vi "Lab Panel V4.91.vi"() -> ()   [LabVIEW 2013] (continued)
                    n1115 = Unbundle(w2166) -> ("CYCLES"=w2157:dbl, "T-RISE mins"=w2163:dbl)  [unwired: 3 out]
                    n1116 = case shown="\"T-RISE TEST\"" w2164 {
                      tunnel: w2163 -> [_ _ w2173]
                      tunnel: [w2168 w2170 w2173] -> w2162
                      tunnel: w2157 -> [w2168 w2170 _]
                      tunnel: ["CHART PASS" "CYCLE PASS" "T-RISE PASS"] -> w2161
                      frame "CHART TEST", Default {
                      }
                      frame "CYCLE TEST" {
                      }
                      frame "T-RISE TEST" {
                      }
                    }
                    n1117 = Increment(x=w2157) -> (x+1=w2158:dbl)
                    n1118 = Greater Or Equal?(x=w2165, y=w2158) -> (x >= y?=w2167:bool)
                    n1119 = case shown="True" w2167 {
                      tunnel: w2162 -> [w2177 _]
                      tunnel: w2161 -> [w2176 _]
                      tunnel: w2160 -> [w2175 _]
                      tunnel: w2159 -> [w2174 _]
                      frame True {
                        n1120 = stacked-sequence {
                          tunnel: w2177 -> [w2181 _]
                          tunnel: w2176 -> [w2179 w2185]
                          tunnel: w2175 -> [_ w2188]
                          tunnel: w2174 -> [w2178 _]
                          frame #0 {
                            n1121 = Build Array(w2179) -> (w2182:string[])
                            n1122 = Build Array(w2181) -> (w2180:dbl[])
                            n1123 = TDMS Write(0:w2178, 5:"TEST PASS", 7:w2182, 9:w2180) -> (15:w2184:errorcluster)  [unwired: 2 in, 3 out]
                            n1124 = local write "data file error"(w2184) -> ()
                          }
                          frame #1 {
                            n1125 = Bundle(cluster=w2188, "STATUS"=w2185) -> (w2186:T4)  [unwired: 2 in]
                            n1126 = local write "RESULT LAB02-1"(TRUE) -> ()
                            n1127 = local write "DISP LAB02-1"(w2186) -> ()
                          }
                        }
                      }
                      frame False {
                      }
                    }
                  }
                }
              }
              frame #3 {
                # "LAB02-2"
                n1128 = Less?(x=w2189, y=2) -> (x < y?=w2192:bool)
                n1129 = local read "DISP LAB02-2"() -> (w2194:T4)
                n1130 = Unbundle(w2194) -> ("STATUS"=w2195:string)  [unwired: 2 out]
                n1131 = Equal?(x=w2195, y="RUN") -> (x = y?=w2191:bool)
                n1132 = And(x=w2191, y=w2192) -> (x .and. y?=w2190:bool)
                n1133 = case shown="True" w2190 {
                  tunnel: w2194 -> [_ w2200]
                  tunnel: w2189 -> [_ w2204]
                  frame False {
                  }
                  frame True {
                    n1134 = local read "SET LAB02-2"() -> (w2206:T5)
                    n1135 = local read "TDMS LAB02-2"() -> (w2199:refnum<k34>)
                    n1136 = Unbundle(w2200) -> ("CYCLE"=w2205:dbl)  [unwired: 2 out]
                    n1137 = Unbundle(w2206) -> ("CYCLES"=w2197:dbl, "T-RISE mins"=w2203:dbl)  [unwired: 3 out]
                    n1138 = case shown="\"T-RISE TEST\"" w2204 {
                      tunnel: w2203 -> [_ _ w2213]
                      tunnel: [w2208 w2210 w2213] -> w2202
                      tunnel: w2197 -> [w2208 w2210 _]
                      tunnel: ["CHART PASS" "CYCLE PASS" "T-RISE PASS"] -> w2201
                      frame "CHART TEST", Default {
                      }
                      frame "CYCLE TEST" {
                      }
                      frame "T-RISE TEST" {
                      }
                    }
                    n1139 = Increment(x=w2197) -> (x+1=w2198:dbl)
                    n1140 = Greater Or Equal?(x=w2205, y=w2198) -> (x >= y?=w2207:bool)
                    n1141 = case shown="True" w2207 {
                      tunnel: w2202 -> [w2217 _]
                      tunnel: w2201 -> [w2216 _]
                      tunnel: w2200 -> [w2215 _]
                      tunnel: w2199 -> [w2214 _]
                      frame True {
                        n1142 = stacked-sequence {
                          tunnel: w2217 -> [w2221 _]
                          tunnel: w2216 -> [w2219 w2225]
                          tunnel: w2215 -> [_ w2228]
                          tunnel: w2214 -> [w2218 _]
                          frame #0 {
                            n1143 = Build Array(w2219) -> (w2222:string[])
                            n1144 = Build Array(w2221) -> (w2220:dbl[])
                            n1145 = TDMS Write(0:w2218, 5:"TEST PASS", 7:w2222, 9:w2220) -> (15:w2224:errorcluster)  [unwired: 2 in, 3 out]
                            n1146 = local write "data file error"(w2224) -> ()
                          }
                          frame #1 {
                            n1147 = Bundle(cluster=w2228, "STATUS"=w2225) -> (w2226:T4)  [unwired: 2 in]
                            n1148 = local write "RESULT LAB02-2"(TRUE) -> ()
                            n1149 = local write "DISP LAB02-2"(w2226) -> ()
                          }
                        }
                      }
                      frame False {
                      }
                    }
                  }
                }
              }
              frame #4 {
                # "LAB03-1"
                n1150 = Less?(x=w2229, y=2) -> (x < y?=w2232:bool)
                n1151 = local read "DISP LAB03-1"() -> (w2234:T4)
                n1152 = Unbundle(w2234) -> ("STATUS"=w2235:string)  [unwired: 2 out]
                n1153 = Equal?(x=w2235, y="RUN") -> (x = y?=w2231:bool)
                n1154 = And(x=w2231, y=w2232) -> (x .and. y?=w2230:bool)
                n1155 = case shown="True" w2230 {
                  tunnel: w2234 -> [_ w2240]
                  tunnel: w2229 -> [_ w2244]
                  frame False {
                  }
                  frame True {
                    n1156 = local read "SET LAB03-1"() -> (w2246:T5)
                    n1157 = local read "TDMS LAB03-1"() -> (w2239:refnum<k34>)
                    n1158 = Unbundle(w2240) -> ("CYCLE"=w2245:dbl)  [unwired: 2 out]
                    n1159 = Unbundle(w2246) -> ("CYCLES"=w2237:dbl, "T-RISE mins"=w2243:dbl)  [unwired: 3 out]
                    n1160 = case shown="\"T-RISE TEST\"" w2244 {
                      tunnel: w2243 -> [_ _ w2253]
                      tunnel: [w2248 w2250 w2253] -> w2242
                      tunnel: w2237 -> [w2248 w2250 _]
                      tunnel: ["CHART PASS" "CYCLE PASS" "T-RISE PASS"] -> w2241
                      frame "CHART TEST", Default {
                      }
                      frame "CYCLE TEST" {
                      }
                      frame "T-RISE TEST" {
                      }
                    }
                    n1161 = Increment(x=w2237) -> (x+1=w2238:dbl)
                    n1162 = Greater Or Equal?(x=w2245, y=w2238) -> (x >= y?=w2247:bool)
                    n1163 = case shown="True" w2247 {
                      tunnel: w2242 -> [w2257 _]
                      tunnel: w2241 -> [w2256 _]
                      tunnel: w2240 -> [w2255 _]
                      tunnel: w2239 -> [w2254 _]
                      frame True {
                        n1164 = stacked-sequence {
                          tunnel: w2257 -> [w2261 _]
                          tunnel: w2256 -> [w2259 w2265]
                          tunnel: w2255 -> [_ w2268]
                          tunnel: w2254 -> [w2258 _]
                          frame #0 {
                            n1165 = Build Array(w2259) -> (w2262:string[])
                            n1166 = Build Array(w2261) -> (w2260:dbl[])
                            n1167 = TDMS Write(0:w2258, 5:"TEST PASS", 7:w2262, 9:w2260) -> (15:w2264:errorcluster)  [unwired: 2 in, 3 out]
                            n1168 = local write "data file error"(w2264) -> ()
                          }
                          frame #1 {
                            n1169 = Bundle(cluster=w2268, "STATUS"=w2265) -> (w2266:T4)  [unwired: 2 in]
                            n1170 = local write "RESULT LAB03-1"(TRUE) -> ()
                            n1171 = local write "DISP LAB03-1"(w2266) -> ()
                          }
                        }
                      }
                      frame False {
                      }
                    }
                  }
                }
              }
              frame #5 {
                # "LAB03-2"
                n1172 = Less?(x=w2269, y=2) -> (x < y?=w2272:bool)
                n1173 = local read "DISP LAB03-2"() -> (w2274:T4)
                n1174 = Unbundle(w2274) -> ("STATUS"=w2275:string)  [unwired: 2 out]
                n1175 = Equal?(x=w2275, y="RUN") -> (x = y?=w2271:bool)
                n1176 = And(x=w2271, y=w2272) -> (x .and. y?=w2270:bool)
                n1177 = case shown="True" w2270 {
                  tunnel: w2274 -> [_ w2280]
                  tunnel: w2269 -> [_ w2284]
                  frame False {
                  }
                  frame True {
                    n1178 = local read "SET LAB03-2"() -> (w2286:T5)
                    n1179 = local read "TDMS LAB03-2"() -> (w2279:refnum<k34>)
                    n1180 = Unbundle(w2280) -> ("CYCLE"=w2285:dbl)  [unwired: 2 out]
                    n1181 = Unbundle(w2286) -> ("CYCLES"=w2277:dbl, "T-RISE mins"=w2283:dbl)  [unwired: 3 out]
                    n1182 = case shown="\"T-RISE TEST\"" w2284 {
                      tunnel: w2283 -> [_ _ w2293]
                      tunnel: [w2288 w2290 w2293] -> w2282
                      tunnel: w2277 -> [w2288 w2290 _]
                      tunnel: ["CHART PASS" "CYCLE PASS" "T-RISE PASS"] -> w2281
                      frame "CHART TEST", Default {
                      }
                      frame "CYCLE TEST" {
                      }
                      frame "T-RISE TEST" {
                      }
                    }
                    n1183 = Increment(x=w2277) -> (x+1=w2278:dbl)
                    n1184 = Greater Or Equal?(x=w2285, y=w2278) -> (x >= y?=w2287:bool)
                    n1185 = case shown="True" w2287 {
                      tunnel: w2282 -> [w2297 _]
                      tunnel: w2281 -> [w2296 _]
                      tunnel: w2280 -> [w2295 _]
                      tunnel: w2279 -> [w2294 _]
                      frame True {
                        n1186 = stacked-sequence {
                          tunnel: w2297 -> [w2301 _]
                          tunnel: w2296 -> [w2299 w2305]
                          tunnel: w2295 -> [_ w2308]
                          tunnel: w2294 -> [w2298 _]
                          frame #0 {
                            n1187 = Build Array(w2299) -> (w2302:string[])
                            n1188 = Build Array(w2301) -> (w2300:dbl[])
                            n1189 = TDMS Write(0:w2298, 5:"TEST PASS", 7:w2302, 9:w2300) -> (15:w2304:errorcluster)  [unwired: 2 in, 3 out]
                            n1190 = local write "data file error"(w2304) -> ()
                          }
                          frame #1 {
                            n1191 = Bundle(cluster=w2308, "STATUS"=w2305) -> (w2306:T4)  [unwired: 2 in]
                            n1192 = local write "RESULT LAB03-2"(TRUE) -> ()
                            n1193 = local write "DISP LAB03-2"(w2306) -> ()
                          }
                        }
                      }
                      frame False {
                      }
                    }
                  }
                }
              }
              frame #6 {
                # "LAB04-1"
                n1194 = Less?(x=w2309, y=2) -> (x < y?=w2312:bool)
                n1195 = local read "DISP LAB04-1"() -> (w2314:T4)
                n1196 = Unbundle(w2314) -> ("STATUS"=w2315:string)  [unwired: 2 out]
                n1197 = Equal?(x=w2315, y="RUN") -> (x = y?=w2311:bool)
                n1198 = And(x=w2311, y=w2312) -> (x .and. y?=w2310:bool)
                n1199 = case shown="True" w2310 {
                  tunnel: w2314 -> [_ w2320]
                  tunnel: w2309 -> [_ w2324]
                  frame False {
                  }
                  frame True {
                    n1200 = local read "SET LAB04-1"() -> (w2326:T5)
                    n1201 = local read "TDMS LAB04-1"() -> (w2319:refnum<k34>)
                    n1202 = Unbundle(w2320) -> ("CYCLE"=w2325:dbl)  [unwired: 2 out]
                    n1203 = Unbundle(w2326) -> ("CYCLES"=w2317:dbl, "T-RISE mins"=w2323:dbl)  [unwired: 3 out]
                    n1204 = case shown="\"T-RISE TEST\"" w2324 {
                      tunnel: w2323 -> [_ _ w2333]
                      tunnel: [w2328 w2330 w2333] -> w2322
                      tunnel: w2317 -> [w2328 w2330 _]
                      tunnel: ["CHART PASS" "CYCLE PASS" "T-RISE PASS"] -> w2321
                      frame "CHART TEST", Default {
                      }
                      frame "CYCLE TEST" {
                      }
                      frame "T-RISE TEST" {
                      }
                    }
                    n1205 = Increment(x=w2317) -> (x+1=w2318:dbl)
                    n1206 = Greater Or Equal?(x=w2325, y=w2318) -> (x >= y?=w2327:bool)
                    n1207 = case shown="True" w2327 {
                      tunnel: w2322 -> [w2337 _]
                      tunnel: w2321 -> [w2336 _]
                      tunnel: w2320 -> [w2335 _]
                      tunnel: w2319 -> [w2334 _]
                      frame True {
                        n1208 = stacked-sequence {
                          tunnel: w2337 -> [w2341 _]
                          tunnel: w2336 -> [w2339 w2345]
                          tunnel: w2335 -> [_ w2348]
                          tunnel: w2334 -> [w2338 _]
                          frame #0 {
                            n1209 = Build Array(w2339) -> (w2342:string[])
                            n1210 = Build Array(w2341) -> (w2340:dbl[])
                            n1211 = TDMS Write(0:w2338, 5:"TEST PASS", 7:w2342, 9:w2340) -> (15:w2344:errorcluster)  [unwired: 2 in, 3 out]
                            n1212 = local write "data file error"(w2344) -> ()
                          }
                          frame #1 {
                            n1213 = Bundle(cluster=w2348, "STATUS"=w2345) -> (w2346:T4)  [unwired: 2 in]
                            n1214 = local write "RESULT LAB04-1"(TRUE) -> ()
                            n1215 = local write "DISP LAB04-1"(w2346) -> ()
                          }
                        }
                      }
                      frame False {
                      }
                    }
                  }
                }
              }
              frame #7 {
                # "LAB04-2"
                n1216 = Less?(x=w2349, y=2) -> (x < y?=w2352:bool)
                n1217 = local read "DISP LAB04-2"() -> (w2354:T4)
                n1218 = Unbundle(w2354) -> ("STATUS"=w2355:string)  [unwired: 2 out]
                n1219 = Equal?(x=w2355, y="RUN") -> (x = y?=w2351:bool)
                n1220 = And(x=w2351, y=w2352) -> (x .and. y?=w2350:bool)
                n1221 = case shown="True" w2350 {
                  tunnel: w2354 -> [_ w2360]
                  tunnel: w2349 -> [_ w2364]
                  frame False {
                  }
                  frame True {
                    n1222 = local read "SET LAB04-2"() -> (w2366:T5)
                    n1223 = local read "TDMS LAB04-2"() -> (w2359:refnum<k34>)
                    n1224 = Unbundle(w2360) -> ("CYCLE"=w2365:dbl)  [unwired: 2 out]
                    n1225 = Unbundle(w2366) -> ("CYCLES"=w2357:dbl, "T-RISE mins"=w2363:dbl)  [unwired: 3 out]
                    n1226 = case shown="\"T-RISE TEST\"" w2364 {
                      tunnel: w2363 -> [_ _ w2373]
                      tunnel: [w2368 w2370 w2373] -> w2362
                      tunnel: w2357 -> [w2368 w2370 _]
                      tunnel: ["CHART PASS" "CYCLE PASS" "T-RISE PASS"] -> w2361
                      frame "CHART TEST", Default {
                      }
                      frame "CYCLE TEST" {
                      }
                      frame "T-RISE TEST" {
                      }
                    }
                    n1227 = Increment(x=w2357) -> (x+1=w2358:dbl)
                    n1228 = Greater Or Equal?(x=w2365, y=w2358) -> (x >= y?=w2367:bool)
                    n1229 = case shown="True" w2367 {
                      tunnel: w2362 -> [w2377 _]
                      tunnel: w2361 -> [w2376 _]
                      tunnel: w2360 -> [w2375 _]
                      tunnel: w2359 -> [w2374 _]
                      frame True {
                        n1230 = stacked-sequence {
                          tunnel: w2377 -> [w2381 _]
                          tunnel: w2376 -> [w2379 w2385]
                          tunnel: w2375 -> [_ w2388]
                          tunnel: w2374 -> [w2378 _]
                          frame #0 {
                            n1231 = Build Array(w2379) -> (w2382:string[])
                            n1232 = Build Array(w2381) -> (w2380:dbl[])
                            n1233 = TDMS Write(0:w2378, 5:"TEST PASS", 7:w2382, 9:w2380) -> (15:w2384:errorcluster)  [unwired: 2 in, 3 out]
                            n1234 = local write "data file error"(w2384) -> ()
                          }
                          frame #1 {
                            n1235 = Bundle(cluster=w2388, "STATUS"=w2385) -> (w2386:T4)  [unwired: 2 in]
                            n1236 = local write "RESULT LAB04-2"(TRUE) -> ()
                            n1237 = local write "DISP LAB04-2"(w2386) -> ()
                          }
                        }
                      }
                      frame False {
                      }
                    }
                  }
                }
              }
              frame #8 {
                # "LAB05-1"
                n1238 = Less?(x=w2389, y=2) -> (x < y?=w2392:bool)
                n1239 = local read "DISP LAB05-1"() -> (w2394:T4)
                n1240 = Unbundle(w2394) -> ("STATUS"=w2395:string)  [unwired: 2 out]
                n1241 = Equal?(x=w2395, y="RUN") -> (x = y?=w2391:bool)
                n1242 = And(x=w2391, y=w2392) -> (x .and. y?=w2390:bool)
                n1243 = case shown="True" w2390 {
                  tunnel: w2394 -> [_ w2400]
                  tunnel: w2389 -> [_ w2404]
                  frame False {
                  }
                  frame True {
                    n1244 = local read "SET LAB05-1"() -> (w2406:T5)
                    n1245 = local read "TDMS LAB05-1"() -> (w2399:refnum<k34>)
                    n1246 = Unbundle(w2400) -> ("CYCLE"=w2405:dbl)  [unwired: 2 out]
                    n1247 = Unbundle(w2406) -> ("CYCLES"=w2397:dbl, "T-RISE mins"=w2403:dbl)  [unwired: 3 out]
                    n1248 = case shown="\"T-RISE TEST\"" w2404 {
                      tunnel: w2403 -> [_ _ w2413]
                      tunnel: [w2408 w2410 w2413] -> w2402
                      tunnel: w2397 -> [w2408 w2410 _]
                      tunnel: ["CHART PASS" "CYCLE PASS" "T-RISE PASS"] -> w2401
                      frame "CHART TEST", Default {
                      }
                      frame "CYCLE TEST" {
                      }
                      frame "T-RISE TEST" {
                      }
                    }
                    n1249 = Increment(x=w2397) -> (x+1=w2398:dbl)
                    n1250 = Greater Or Equal?(x=w2405, y=w2398) -> (x >= y?=w2407:bool)
                    n1251 = case shown="True" w2407 {
                      tunnel: w2402 -> [w2417 _]
                      tunnel: w2401 -> [w2416 _]
                      tunnel: w2400 -> [w2415 _]
                      tunnel: w2399 -> [w2414 _]
                      frame True {
                        n1252 = stacked-sequence {
                          tunnel: w2417 -> [w2421 _]
                          tunnel: w2416 -> [w2419 w2425]
                          tunnel: w2415 -> [_ w2428]
                          tunnel: w2414 -> [w2418 _]
                          frame #0 {
                            n1253 = Build Array(w2419) -> (w2422:string[])
                            n1254 = Build Array(w2421) -> (w2420:dbl[])
                            n1255 = TDMS Write(0:w2418, 5:"TEST PASS", 7:w2422, 9:w2420) -> (15:w2424:errorcluster)  [unwired: 2 in, 3 out]
                            n1256 = local write "data file error"(w2424) -> ()
                          }
                          frame #1 {
                            n1257 = Bundle(cluster=w2428, "STATUS"=w2425) -> (w2426:T4)  [unwired: 2 in]
                            n1258 = local write "RESULT LAB05-1"(TRUE) -> ()
                            n1259 = local write "DISP LAB05-1"(w2426) -> ()
                          }
                        }
                      }
                      frame False {
                      }
                    }
                  }
                }
              }
              frame #9 {
                # "LAB05-2"
                n1260 = Less?(x=w2429, y=2) -> (x < y?=w2432:bool)
                n1261 = local read "DISP LAB05-2"() -> (w2434:T4)
                n1262 = Unbundle(w2434) -> ("STATUS"=w2435:string)  [unwired: 2 out]
                n1263 = Equal?(x=w2435, y="RUN") -> (x = y?=w2431:bool)
                n1264 = And(x=w2431, y=w2432) -> (x .and. y?=w2430:bool)
                n1265 = case shown="True" w2430 {
                  tunnel: w2434 -> [_ w2440]
                  tunnel: w2429 -> [_ w2444]
                  frame False {
                  }
                  frame True {
                    n1266 = local read "SET LAB05-2"() -> (w2446:T5)
                    n1267 = local read "TDMS LAB05-2"() -> (w2439:refnum<k34>)
                    n1268 = Unbundle(w2440) -> ("CYCLE"=w2445:dbl)  [unwired: 2 out]
                    n1269 = Unbundle(w2446) -> ("CYCLES"=w2437:dbl, "T-RISE mins"=w2443:dbl)  [unwired: 3 out]
                    n1270 = case shown="\"T-RISE TEST\"" w2444 {
                      tunnel: w2443 -> [_ _ w2453]
                      tunnel: [w2448 w2450 w2453] -> w2442
                      tunnel: w2437 -> [w2448 w2450 _]
                      tunnel: ["CHART PASS" "CYCLE PASS" "T-RISE PASS"] -> w2441
                      frame "CHART TEST", Default {
                      }
                      frame "CYCLE TEST" {
                      }
                      frame "T-RISE TEST" {
                      }
                    }
                    n1271 = Increment(x=w2437) -> (x+1=w2438:dbl)
                    n1272 = Greater Or Equal?(x=w2445, y=w2438) -> (x >= y?=w2447:bool)
                    n1273 = case shown="True" w2447 {
                      tunnel: w2442 -> [w2457 _]
                      tunnel: w2441 -> [w2456 _]
                      tunnel: w2440 -> [w2455 _]
                      tunnel: w2439 -> [w2454 _]
                      frame True {
                        n1274 = stacked-sequence {
                          tunnel: w2457 -> [w2461 _]
                          tunnel: w2456 -> [w2459 w2465]
                          tunnel: w2455 -> [_ w2468]
                          tunnel: w2454 -> [w2458 _]
                          frame #0 {
                            n1275 = Build Array(w2459) -> (w2462:string[])
                            n1276 = Build Array(w2461) -> (w2460:dbl[])
                            n1277 = TDMS Write(0:w2458, 5:"TEST PASS", 7:w2462, 9:w2460) -> (15:w2464:errorcluster)  [unwired: 2 in, 3 out]
                            n1278 = local write "data file error"(w2464) -> ()
                          }
                          frame #1 {
                            n1279 = Bundle(cluster=w2468, "STATUS"=w2465) -> (w2466:T4)  [unwired: 2 in]
                            n1280 = local write "RESULT LAB05-2"(TRUE) -> ()
                            n1281 = local write "DISP LAB05-2"(w2466) -> ()
                          }
                        }
                      }
                      frame False {
                      }
                    }
                  }
                }
              }
            }
          }
          frame #5 {
            # "check if test cycles reached for temperature rise test"
            n1282 = stacked-sequence {
              tunnel: w2498 -> [_ _ _ _ _ _ _ _ _ _]
              tunnel: w2497 -> [_ _ _ _ _ _ _ _ _ _]
              tunnel: w2496 -> [_ _ _ _ _ _ _ _ _ _]
              tunnel: w2495 -> [_ _ _ _ _ _ _ _ _ _]
              tunnel: w2494 -> [_ _ _ _ _ _ _ _ _ _]
              tunnel: w2493 -> [_ _ _ _ _ _ _ _ _ _]
              tunnel: w2492 -> [_ _ _ _ _ _ _ _ _ _]
              tunnel: w2491 -> [_ _ _ _ _ _ _ _ _ _]
              tunnel: w2490 -> [_ _ _ _ _ _ _ _ _ _]
              tunnel: w2489 -> [_ _ _ _ _ _ _ _ _ _]
              tunnel: w2488 -> [w2504 _ _ _ _ _ _ _ _ _]
              tunnel: w2478 -> [w2499 _ _ _ _ _ _ _ _ _]
              tunnel: w2487 -> [_ w2530 _ _ _ _ _ _ _ _]
              tunnel: w2486 -> [_ _ w2560 _ _ _ _ _ _ _]
              tunnel: w2485 -> [_ _ _ w2590 _ _ _ _ _ _]
              tunnel: w2484 -> [_ _ _ _ w2620 _ _ _ _ _]
              tunnel: w2483 -> [_ _ _ _ _ w2650 _ _ _ _]
              tunnel: w2482 -> [_ _ _ _ _ _ w2680 _ _ _]
              tunnel: w2481 -> [_ _ _ _ _ _ _ w2710 _ _]
              tunnel: w2480 -> [_ _ _ _ _ _ _ _ w2740 _]
              tunnel: w2479 -> [_ _ _ _ _ _ _ _ _ w2770]
              tunnel: w2477 -> [_ w2529 _ _ _ _ _ _ _ _]
              tunnel: w2476 -> [_ _ w2559 _ _ _ _ _ _ _]
              tunnel: w2475 -> [_ _ _ w2589 _ _ _ _ _ _]
              tunnel: w2474 -> [_ _ _ _ w2619 _ _ _ _ _]
              tunnel: w2473 -> [_ _ _ _ _ w2649 _ _ _ _]
              tunnel: w2472 -> [_ _ _ _ _ _ w2679 _ _ _]
              tunnel: w2471 -> [_ _ _ _ _ _ _ w2709 _ _]
              tunnel: w2470 -> [_ _ _ _ _ _ _ _ w2739 _]
              tunnel: w2469 -> [_ _ _ _ _ _ _ _ _ w2769]
              frame #0 {
                # "LAB01-1"
                n1283 = Equal?(x=w2504, y=2) -> (x = y?=w2502:bool)
                n1284 = local read "DISP LAB01-1"() -> (w2505:T4)
                n1285 = Unbundle(w2505) -> ("STATUS"=w2506:string)  [unwired: 2 out]
                n1286 = Equal?(x=w2506, y="RUN") -> (x = y?=w2501:bool)
                n1287 = And(x=w2501, y=w2502) -> (x .and. y?=w2500:bool)
                n1288 = case shown="True" w2500 {
                  tunnel: w2505 -> [_ w2509]
                  tunnel: w2499 -> [_ w2512]
                  frame False {
                  }
                  frame True {
                    n1289 = local read "SET LAB01-1"() -> (w2511:T5)
                    n1290 = local read "TDMS LAB01-1"() -> (w2508:refnum<k34>)
                    n1291 = Unbundle(w2509) -> ("CYCLE"=w2513:dbl)  [unwired: 2 out]
                    n1292 = Unbundle(w2511) -> ("T-RISE mins"=w2510:dbl)  [unwired: 4 out]
                    n1293 = Greater Or Equal?(x=w2513, y=w2512) -> (x >= y?=w2514:bool)
                    n1294 = case shown="True" w2514 {
                      tunnel: w2510 -> [w2517 _]
                      tunnel: w2509 -> [w2516 _]
                      tunnel: w2508 -> [w2515 _]
                      frame True {
                        n1295 = stacked-sequence {
                          tunnel: w2517 -> [w2520 _]
                          tunnel: w2516 -> [_ w2525]
                          tunnel: w2515 -> [w2518 _]
                          frame #0 {
                            n1296 = Build Array("T-RISE") -> (w2522:string[])
                            n1297 = Build Array(w2520) -> (w2521:dbl[])
                            n1298 = TDMS Write(0:w2518, 5:"TEST PASS", 7:w2522, 9:w2521) -> (15:w2524:errorcluster)  [unwired: 2 in, 3 out]
                            n1299 = local write "data file error"(w2524) -> ()
                          }
                          frame #1 {
                            n1300 = Bundle(cluster=w2525, "STATUS"="T-RISE PASS") -> (w2527:T4)  [unwired: 2 in]
                            n1301 = local write "RESULT LAB01-1"(TRUE) -> ()
                            n1302 = local write "DISP LAB01-1"(w2527) -> ()
                          }
                        }
                      }
                      frame False {
                      }
                    }
                  }
                }
              }
              frame #1 {
                # "LAB01-2"
                n1303 = Equal?(x=w2530, y=2) -> (x = y?=w2533:bool)
                n1304 = local read "DISP LAB01-2"() -> (w2535:T4)
                n1305 = Unbundle(w2535) -> ("STATUS"=w2536:string)  [unwired: 2 out]
                n1306 = Equal?(x=w2536, y="RUN") -> (x = y?=w2532:bool)
                n1307 = And(x=w2532, y=w2533) -> (x .and. y?=w2531:bool)
                n1308 = case shown="True" w2531 {
                  tunnel: w2535 -> [_ w2539]
                  tunnel: w2529 -> [_ w2542]
                  frame False {
                  }
                  frame True {
                    n1309 = local read "SET LAB01-2"() -> (w2541:T5)
                    n1310 = local read "TDMS LAB01-2"() -> (w2538:refnum<k34>)
                    n1311 = Unbundle(w2539) -> ("CYCLE"=w2543:dbl)  [unwired: 2 out]
                    n1312 = Unbundle(w2541) -> ("T-RISE mins"=w2540:dbl)  [unwired: 4 out]
                    n1313 = Greater Or Equal?(x=w2543, y=w2542) -> (x >= y?=w2544:bool)
                    n1314 = case shown="True" w2544 {
                      tunnel: w2540 -> [w2547 _]
                      tunnel: w2539 -> [w2546 _]
                      tunnel: w2538 -> [w2545 _]
                      frame True {
                        n1315 = stacked-sequence {
                          tunnel: w2547 -> [w2550 _]
                          tunnel: w2546 -> [_ w2555]
                          tunnel: w2545 -> [w2548 _]
                          frame #0 {
                            n1316 = Build Array("T-RISE") -> (w2552:string[])
                            n1317 = Build Array(w2550) -> (w2551:dbl[])
                            n1318 = TDMS Write(0:w2548, 5:"TEST PASS", 7:w2552, 9:w2551) -> (15:w2554:errorcluster)  [unwired: 2 in, 3 out]
                            n1319 = local write "data file error"(w2554) -> ()
                          }
                          frame #1 {
                            n1320 = Bundle(cluster=w2555, "STATUS"="T-RISE PASS") -> (w2557:T4)  [unwired: 2 in]
                            n1321 = local write "RESULT LAB01-2"(TRUE) -> ()
                            n1322 = local write "DISP LAB01-2"(w2557) -> ()
                          }
                        }
                      }
                      frame False {
                      }
                    }
                  }
                }
              }
              frame #2 {
                # "LAB02-1"
                n1323 = Equal?(x=w2560, y=2) -> (x = y?=w2563:bool)
                n1324 = local read "DISP LAB02-1"() -> (w2565:T4)
                n1325 = Unbundle(w2565) -> ("STATUS"=w2566:string)  [unwired: 2 out]
                n1326 = Equal?(x=w2566, y="RUN") -> (x = y?=w2562:bool)
                n1327 = And(x=w2562, y=w2563) -> (x .and. y?=w2561:bool)
                n1328 = case shown="True" w2561 {
                  tunnel: w2565 -> [_ w2569]
                  tunnel: w2559 -> [_ w2572]
                  frame False {
                  }
                  frame True {
                    n1329 = local read "SET LAB02-1"() -> (w2571:T5)
                    n1330 = local read "TDMS LAB02-1"() -> (w2568:refnum<k34>)
                    n1331 = Unbundle(w2569) -> ("CYCLE"=w2573:dbl)  [unwired: 2 out]
                    n1332 = Unbundle(w2571) -> ("T-RISE mins"=w2570:dbl)  [unwired: 4 out]
                    n1333 = Greater Or Equal?(x=w2573, y=w2572) -> (x >= y?=w2574:bool)
                    n1334 = case shown="True" w2574 {
                      tunnel: w2570 -> [w2577 _]
                      tunnel: w2569 -> [w2576 _]
                      tunnel: w2568 -> [w2575 _]
                      frame True {
                        n1335 = stacked-sequence {
                          tunnel: w2577 -> [w2580 _]
                          tunnel: w2576 -> [_ w2585]
                          tunnel: w2575 -> [w2578 _]
                          frame #0 {
                            n1336 = Build Array("T-RISE") -> (w2582:string[])
                            n1337 = Build Array(w2580) -> (w2581:dbl[])
                            n1338 = TDMS Write(0:w2578, 5:"TEST PASS", 7:w2582, 9:w2581) -> (15:w2584:errorcluster)  [unwired: 2 in, 3 out]
                            n1339 = local write "data file error"(w2584) -> ()
                          }
                          frame #1 {
                            n1340 = Bundle(cluster=w2585, "STATUS"="T-RISE PASS") -> (w2587:T4)  [unwired: 2 in]
                            n1341 = local write "RESULT LAB02-1"(TRUE) -> ()
                            n1342 = local write "DISP LAB02-1"(w2587) -> ()
                          }
                        }
                      }
                      frame False {
                      }
                    }
                  }
                }
              }
              frame #3 {
                # "LAB02-2"
                n1343 = Equal?(x=w2590, y=2) -> (x = y?=w2593:bool)
                n1344 = local read "DISP LAB02-2"() -> (w2595:T4)
                n1345 = Unbundle(w2595) -> ("STATUS"=w2596:string)  [unwired: 2 out]
                n1346 = Equal?(x=w2596, y="RUN") -> (x = y?=w2592:bool)
                n1347 = And(x=w2592, y=w2593) -> (x .and. y?=w2591:bool)
                n1348 = case shown="True" w2591 {
                  tunnel: w2595 -> [_ w2599]
                  tunnel: w2589 -> [_ w2602]
                  frame False {
                  }
                  frame True {
                    n1349 = local read "SET LAB02-2"() -> (w2601:T5)
                    n1350 = local read "TDMS LAB02-2"() -> (w2598:refnum<k34>)
                    n1351 = Unbundle(w2599) -> ("CYCLE"=w2603:dbl)  [unwired: 2 out]
                    n1352 = Unbundle(w2601) -> ("T-RISE mins"=w2600:dbl)  [unwired: 4 out]
                    n1353 = Greater Or Equal?(x=w2603, y=w2602) -> (x >= y?=w2604:bool)
                    n1354 = case shown="True" w2604 {
                      tunnel: w2600 -> [w2607 _]
                      tunnel: w2599 -> [w2606 _]
                      tunnel: w2598 -> [w2605 _]
                      frame True {
                        n1355 = stacked-sequence {
                          tunnel: w2607 -> [w2610 _]
                          tunnel: w2606 -> [_ w2615]
                          tunnel: w2605 -> [w2608 _]
                          frame #0 {
                            n1356 = Build Array("T-RISE") -> (w2612:string[])
                            n1357 = Build Array(w2610) -> (w2611:dbl[])
                            n1358 = TDMS Write(0:w2608, 5:"TEST PASS", 7:w2612, 9:w2611) -> (15:w2614:errorcluster)  [unwired: 2 in, 3 out]
                            n1359 = local write "data file error"(w2614) -> ()
                          }
                          frame #1 {
                            n1360 = Bundle(cluster=w2615, "STATUS"="T-RISE PASS") -> (w2617:T4)  [unwired: 2 in]
                            n1361 = local write "RESULT LAB02-2"(TRUE) -> ()
                            n1362 = local write "DISP LAB02-2"(w2617) -> ()
                          }
                        }
                      }
                      frame False {
                      }
                    }
                  }
                }
              }
              frame #4 {
                # "LAB03-1"
                n1363 = Equal?(x=w2620, y=2) -> (x = y?=w2623:bool)
                n1364 = local read "DISP LAB03-1"() -> (w2625:T4)
                n1365 = Unbundle(w2625) -> ("STATUS"=w2626:string)  [unwired: 2 out]
                n1366 = Equal?(x=w2626, y="RUN") -> (x = y?=w2622:bool)
                n1367 = And(x=w2622, y=w2623) -> (x .and. y?=w2621:bool)
                n1368 = case shown="True" w2621 {
                  tunnel: w2625 -> [_ w2629]
                  tunnel: w2619 -> [_ w2632]
                  frame False {
                  }
                  frame True {
                    n1369 = local read "SET LAB03-1"() -> (w2631:T5)
                    n1370 = local read "TDMS LAB03-1"() -> (w2628:refnum<k34>)
                    n1371 = Unbundle(w2629) -> ("CYCLE"=w2633:dbl)  [unwired: 2 out]
                    n1372 = Unbundle(w2631) -> ("T-RISE mins"=w2630:dbl)  [unwired: 4 out]
                    n1373 = Greater Or Equal?(x=w2633, y=w2632) -> (x >= y?=w2634:bool)
                    n1374 = case shown="True" w2634 {
                      tunnel: w2630 -> [w2637 _]
                      tunnel: w2629 -> [w2636 _]
                      tunnel: w2628 -> [w2635 _]
                      frame True {
                        n1375 = stacked-sequence {
                          tunnel: w2637 -> [w2640 _]
                          tunnel: w2636 -> [_ w2645]
                          tunnel: w2635 -> [w2638 _]
                          frame #0 {
                            n1376 = Build Array("T-RISE") -> (w2642:string[])
                            n1377 = Build Array(w2640) -> (w2641:dbl[])
                            n1378 = TDMS Write(0:w2638, 5:"TEST PASS", 7:w2642, 9:w2641) -> (15:w2644:errorcluster)  [unwired: 2 in, 3 out]
                            n1379 = local write "data file error"(w2644) -> ()
                          }
                          frame #1 {
                            n1380 = Bundle(cluster=w2645, "STATUS"="T-RISE PASS") -> (w2647:T4)  [unwired: 2 in]
                            n1381 = local write "RESULT LAB03-1"(TRUE) -> ()
                            n1382 = local write "DISP LAB03-1"(w2647) -> ()
                          }
                        }
                      }
                      frame False {
                      }
                    }
                  }
                }
              }
              frame #5 {
                # "LAB03-2"
                n1383 = Equal?(x=w2650, y=2) -> (x = y?=w2653:bool)
                n1384 = local read "DISP LAB03-2"() -> (w2655:T4)
                n1385 = Unbundle(w2655) -> ("STATUS"=w2656:string)  [unwired: 2 out]
                n1386 = Equal?(x=w2656, y="RUN") -> (x = y?=w2652:bool)
                n1387 = And(x=w2652, y=w2653) -> (x .and. y?=w2651:bool)
                n1388 = case shown="True" w2651 {
                  tunnel: w2655 -> [_ w2659]
                  tunnel: w2649 -> [_ w2662]
                  frame False {
                  }
                  frame True {
                    n1389 = local read "SET LAB03-2"() -> (w2661:T5)
                    n1390 = local read "TDMS LAB03-2"() -> (w2658:refnum<k34>)
                    n1391 = Unbundle(w2659) -> ("CYCLE"=w2663:dbl)  [unwired: 2 out]
                    n1392 = Unbundle(w2661) -> ("T-RISE mins"=w2660:dbl)  [unwired: 4 out]
                    n1393 = Greater Or Equal?(x=w2663, y=w2662) -> (x >= y?=w2664:bool)
                    n1394 = case shown="True" w2664 {
                      tunnel: w2660 -> [w2667 _]
                      tunnel: w2659 -> [w2666 _]
                      tunnel: w2658 -> [w2665 _]
                      frame True {
                        n1395 = stacked-sequence {
                          tunnel: w2667 -> [w2670 _]
                          tunnel: w2666 -> [_ w2675]
                          tunnel: w2665 -> [w2668 _]
                          frame #0 {
                            n1396 = Build Array("T-RISE") -> (w2672:string[])
                            n1397 = Build Array(w2670) -> (w2671:dbl[])
                            n1398 = TDMS Write(0:w2668, 5:"TEST PASS", 7:w2672, 9:w2671) -> (15:w2674:errorcluster)  [unwired: 2 in, 3 out]
                            n1399 = local write "data file error"(w2674) -> ()
                          }
                          frame #1 {
                            n1400 = Bundle(cluster=w2675, "STATUS"="T-RISE PASS") -> (w2677:T4)  [unwired: 2 in]
                            n1401 = local write "RESULT LAB03-2"(TRUE) -> ()
                            n1402 = local write "DISP LAB03-2"(w2677) -> ()
                          }
                        }
                      }
                      frame False {
                      }
                    }
                  }
                }
              }
              frame #6 {
                # "LAB04-1"
                n1403 = Equal?(x=w2680, y=2) -> (x = y?=w2683:bool)
                n1404 = local read "DISP LAB04-1"() -> (w2685:T4)
                n1405 = Unbundle(w2685) -> ("STATUS"=w2686:string)  [unwired: 2 out]
                n1406 = Equal?(x=w2686, y="RUN") -> (x = y?=w2682:bool)
                n1407 = And(x=w2682, y=w2683) -> (x .and. y?=w2681:bool)
                n1408 = case shown="True" w2681 {
                  tunnel: w2685 -> [_ w2689]
                  tunnel: w2679 -> [_ w2692]
                  frame False {
                  }
                  frame True {
                    n1409 = local read "SET LAB04-1"() -> (w2691:T5)
                    n1410 = local read "TDMS LAB04-1"() -> (w2688:refnum<k34>)
                    n1411 = Unbundle(w2689) -> ("CYCLE"=w2693:dbl)  [unwired: 2 out]
                    n1412 = Unbundle(w2691) -> ("T-RISE mins"=w2690:dbl)  [unwired: 4 out]
                    n1413 = Greater Or Equal?(x=w2693, y=w2692) -> (x >= y?=w2694:bool)
                    n1414 = case shown="True" w2694 {
                      tunnel: w2690 -> [w2697 _]
                      tunnel: w2689 -> [w2696 _]
                      tunnel: w2688 -> [w2695 _]
                      frame True {
                        n1415 = stacked-sequence {
                          tunnel: w2697 -> [w2700 _]
                          tunnel: w2696 -> [_ w2705]
                          tunnel: w2695 -> [w2698 _]
                          frame #0 {
                            n1416 = Build Array("T-RISE") -> (w2702:string[])
                            n1417 = Build Array(w2700) -> (w2701:dbl[])
                            n1418 = TDMS Write(0:w2698, 5:"TEST PASS", 7:w2702, 9:w2701) -> (15:w2704:errorcluster)  [unwired: 2 in, 3 out]
                            n1419 = local write "data file error"(w2704) -> ()
                          }
                          frame #1 {
                            n1420 = Bundle(cluster=w2705, "STATUS"="T-RISE PASS") -> (w2707:T4)  [unwired: 2 in]
                            n1421 = local write "RESULT LAB04-1"(TRUE) -> ()
                            n1422 = local write "DISP LAB04-1"(w2707) -> ()
                          }
                        }
                      }
                      frame False {
                      }
                    }
                  }
                }
              }
              frame #7 {
                # "LAB04-2"
                n1423 = Equal?(x=w2710, y=2) -> (x = y?=w2713:bool)
                n1424 = local read "DISP LAB04-2"() -> (w2715:T4)
                n1425 = Unbundle(w2715) -> ("STATUS"=w2716:string)  [unwired: 2 out]
                n1426 = Equal?(x=w2716, y="RUN") -> (x = y?=w2712:bool)
                n1427 = And(x=w2712, y=w2713) -> (x .and. y?=w2711:bool)
                n1428 = case shown="True" w2711 {
                  tunnel: w2715 -> [_ w2719]
                  tunnel: w2709 -> [_ w2722]
                  frame False {
                  }
                  frame True {
                    n1429 = local read "SET LAB04-2"() -> (w2721:T5)
                    n1430 = local read "TDMS LAB04-2"() -> (w2718:refnum<k34>)
                    n1431 = Unbundle(w2719) -> ("CYCLE"=w2723:dbl)  [unwired: 2 out]
                    n1432 = Unbundle(w2721) -> ("T-RISE mins"=w2720:dbl)  [unwired: 4 out]
                    n1433 = Greater Or Equal?(x=w2723, y=w2722) -> (x >= y?=w2724:bool)
                    n1434 = case shown="True" w2724 {
                      tunnel: w2720 -> [w2727 _]
                      tunnel: w2719 -> [w2726 _]
                      tunnel: w2718 -> [w2725 _]
                      frame True {
                        n1435 = stacked-sequence {
                          tunnel: w2727 -> [w2730 _]
                          tunnel: w2726 -> [_ w2735]
                          tunnel: w2725 -> [w2728 _]
                          frame #0 {
                            n1436 = Build Array("T-RISE") -> (w2732:string[])
                            n1437 = Build Array(w2730) -> (w2731:dbl[])
                            n1438 = TDMS Write(0:w2728, 5:"TEST PASS", 7:w2732, 9:w2731) -> (15:w2734:errorcluster)  [unwired: 2 in, 3 out]
                            n1439 = local write "data file error"(w2734) -> ()
                          }
                          frame #1 {
                            n1440 = Bundle(cluster=w2735, "STATUS"="T-RISE PASS") -> (w2737:T4)  [unwired: 2 in]
                            n1441 = local write "RESULT LAB04-2"(TRUE) -> ()
                            n1442 = local write "DISP LAB04-2"(w2737) -> ()
                          }
                        }
                      }
                      frame False {
                      }
                    }
                  }
                }
              }
              frame #8 {
                # "LAB05-1"
                n1443 = Equal?(x=w2740, y=2) -> (x = y?=w2743:bool)
                n1444 = local read "DISP LAB05-1"() -> (w2745:T4)
                n1445 = Unbundle(w2745) -> ("STATUS"=w2746:string)  [unwired: 2 out]
                n1446 = Equal?(x=w2746, y="RUN") -> (x = y?=w2742:bool)
                n1447 = And(x=w2742, y=w2743) -> (x .and. y?=w2741:bool)
                n1448 = case shown="True" w2741 {
                  tunnel: w2745 -> [_ w2749]
                  tunnel: w2739 -> [_ w2752]
                  frame False {
                  }
                  frame True {
                    n1449 = local read "SET LAB05-1"() -> (w2751:T5)
                    n1450 = local read "TDMS LAB05-1"() -> (w2748:refnum<k34>)
                    n1451 = Unbundle(w2749) -> ("CYCLE"=w2753:dbl)  [unwired: 2 out]
                    n1452 = Unbundle(w2751) -> ("T-RISE mins"=w2750:dbl)  [unwired: 4 out]
                    n1453 = Greater Or Equal?(x=w2753, y=w2752) -> (x >= y?=w2754:bool)
                    n1454 = case shown="True" w2754 {
                      tunnel: w2750 -> [w2757 _]
                      tunnel: w2749 -> [w2756 _]
                      tunnel: w2748 -> [w2755 _]
                      frame True {
                        n1455 = stacked-sequence {
                          tunnel: w2757 -> [w2760 _]
                          tunnel: w2756 -> [_ w2765]
                          tunnel: w2755 -> [w2758 _]
                          frame #0 {
                            n1456 = Build Array("T-RISE") -> (w2762:string[])
                            n1457 = Build Array(w2760) -> (w2761:dbl[])
                            n1458 = TDMS Write(0:w2758, 5:"TEST PASS", 7:w2762, 9:w2761) -> (15:w2764:errorcluster)  [unwired: 2 in, 3 out]
                            n1459 = local write "data file error"(w2764) -> ()
                          }
                          frame #1 {
                            n1460 = Bundle(cluster=w2765, "STATUS"="T-RISE PASS") -> (w2767:T4)  [unwired: 2 in]
                            n1461 = local write "RESULT LAB05-1"(TRUE) -> ()
                            n1462 = local write "DISP LAB05-1"(w2767) -> ()
                          }
                        }
                      }
                      frame False {
                      }
                    }
                  }
                }
              }
              frame #9 {
                # "LAB05-2"
                n1463 = Equal?(x=w2770, y=2) -> (x = y?=w2773:bool)
                n1464 = local read "DISP LAB05-2"() -> (w2775:T4)
                n1465 = Unbundle(w2775) -> ("STATUS"=w2776:string)  [unwired: 2 out]
                n1466 = Equal?(x=w2776, y="RUN") -> (x = y?=w2772:bool)
                n1467 = And(x=w2772, y=w2773) -> (x .and. y?=w2771:bool)
                n1468 = case shown="True" w2771 {
                  tunnel: w2775 -> [_ w2779]
                  tunnel: w2769 -> [_ w2782]
                  frame False {
                  }
                  frame True {
                    n1469 = local read "SET LAB05-2"() -> (w2781:T5)
                    n1470 = local read "TDMS LAB05-2"() -> (w2778:refnum<k34>)
                    n1471 = Unbundle(w2779) -> ("CYCLE"=w2783:dbl)  [unwired: 2 out]
                    n1472 = Unbundle(w2781) -> ("T-RISE mins"=w2780:dbl)  [unwired: 4 out]
                    n1473 = Greater Or Equal?(x=w2783, y=w2782) -> (x >= y?=w2784:bool)
                    n1474 = case shown="True" w2784 {
                      tunnel: w2780 -> [w2787 _]
                      tunnel: w2779 -> [w2786 _]
                      tunnel: w2778 -> [w2785 _]
                      frame True {
                        n1475 = stacked-sequence {
